vi "Analog Sensors.vi"() -> ()   [LabVIEW 2014]
uses:
  <vilib>/eio/EIONode/EIONode.xnode
  <vilib>/rvi/eio/common/nirviEmuTemplateMethod_errors.vi
panel:
  out "5V Reference":fxp<+/-,16,5>
  out "Throttle Percentage":fxp<+/-,33,17>
  out "Throttle Pot (V)":fxp<+/-,16,5>
  out "Rotation Rate (degrees/s)":fxp<+/-,64,33>
  out "Steering Wheel Angle (degrees)":fxp<+/-,48,32>
  out "ticks/count 4":u32
  out "ticks/count 3":u32
  out "ticks/count 2":u32
  out "ticks/count":u32
  in  "stop 2":bool
  out "SpeedZ":fxp<+/-,32,29>
  out "SpeedY":fxp<+/-,32,29>
  out "SpeedX":fxp<+/-,32,29>
  out "AccelZ (G)":fxp<+/-,42,25>
  out "AccelY (G)":fxp<+/-,42,25>
  out "AccelX (G)":fxp<+/-,42,25>
  in  "stop":bool
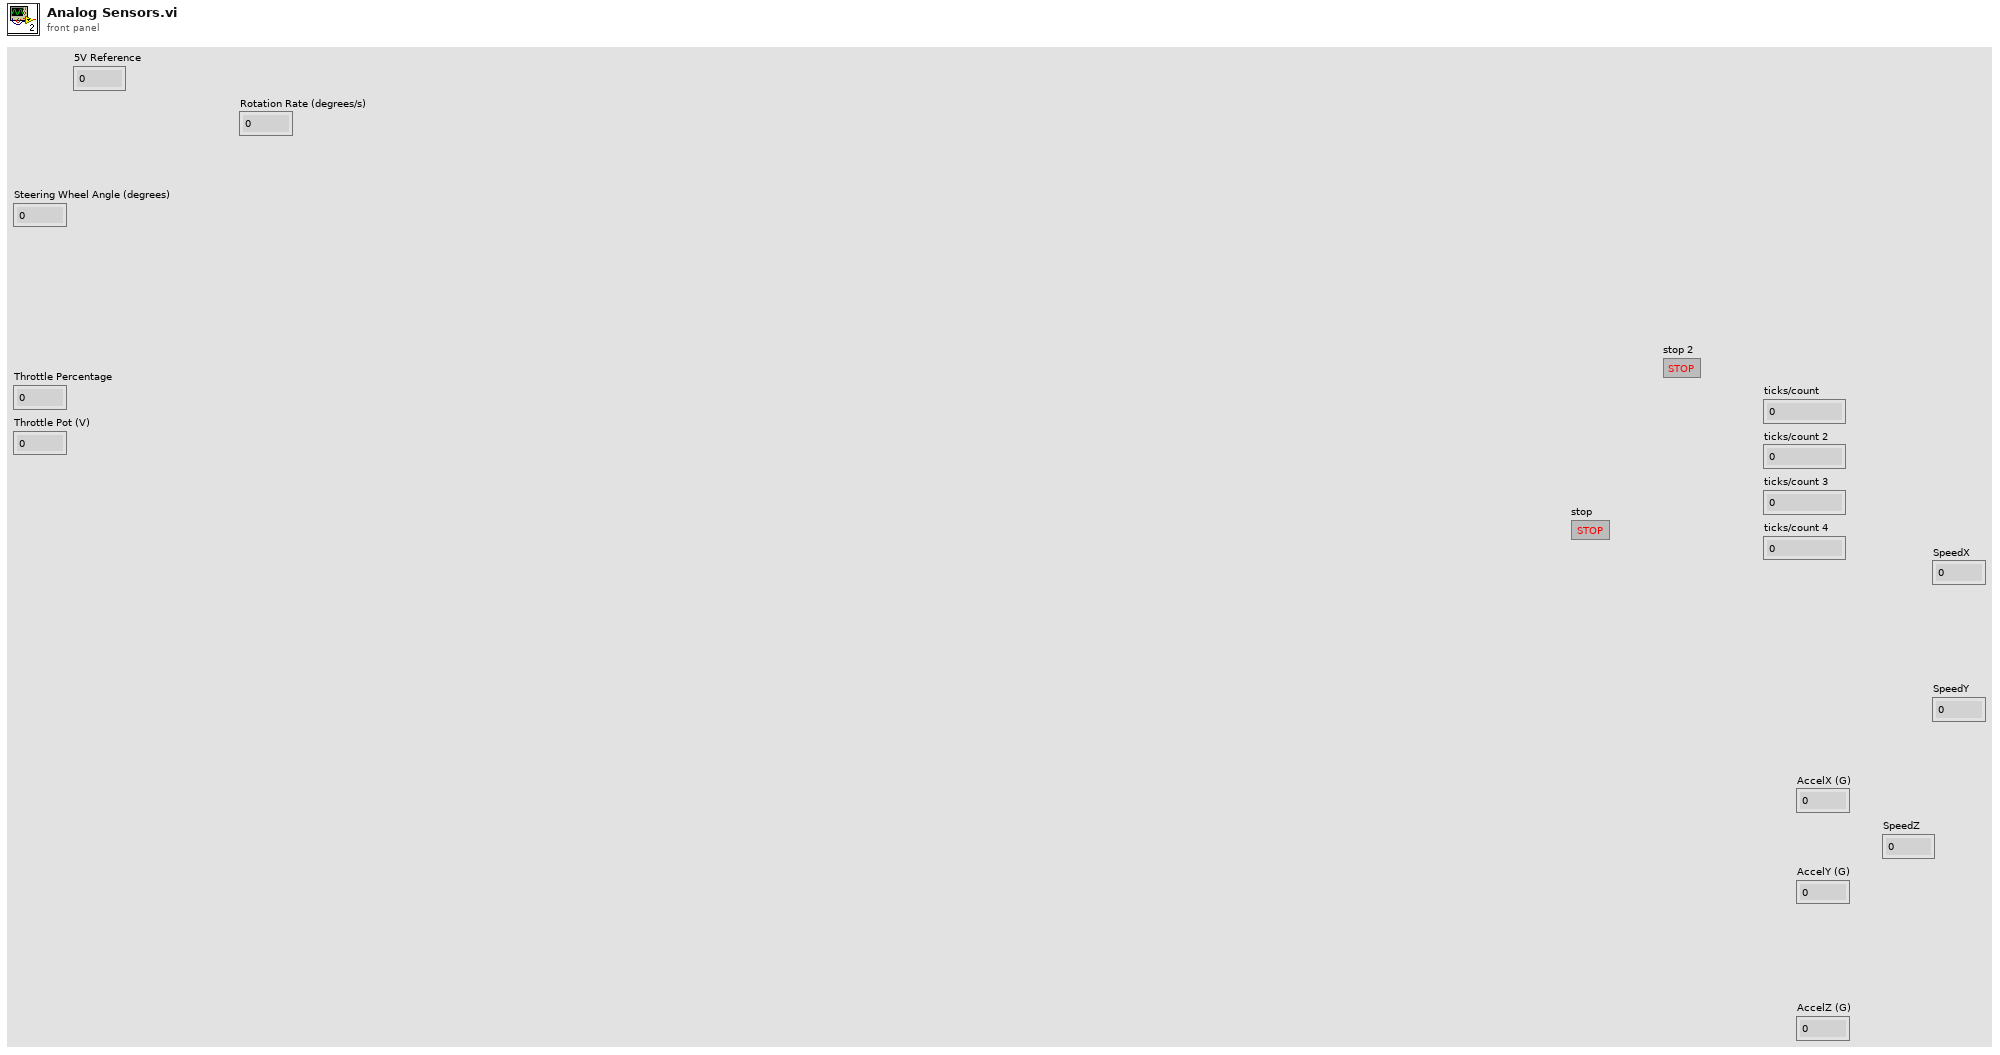
[diagram p1: front panel]
types:
  T1 = enum16{"Wheel Speed 1", "Wheel Speed 2", "Wheel Speed 3", "Wheel Speed 4"}
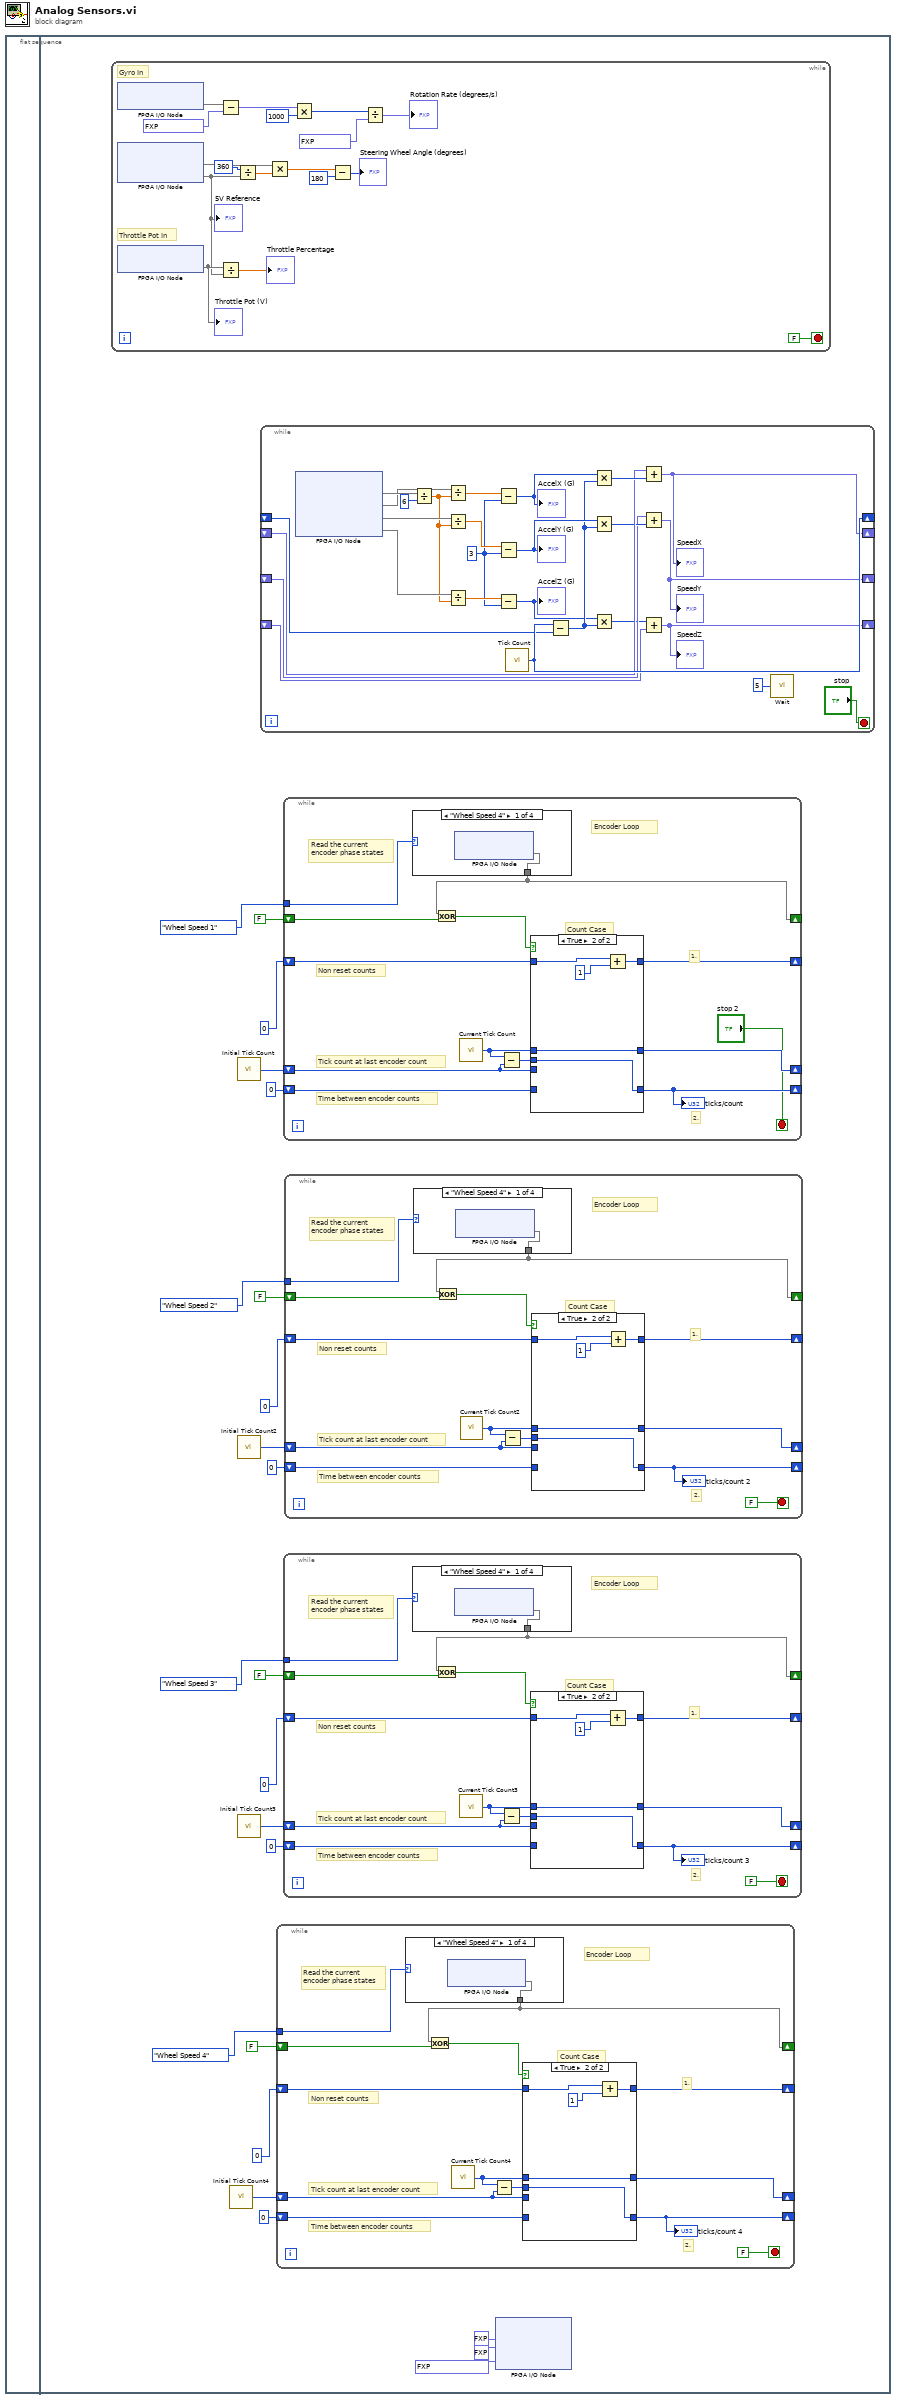
[diagram p0: block diagram]
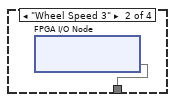
[diagram p2: hidden frame]
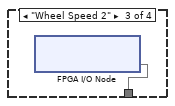
[diagram p3: hidden frame]
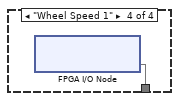
[diagram p4: hidden frame]
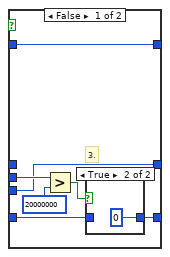
[diagram p5: hidden frame]
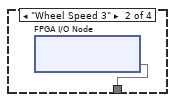
[diagram p7: hidden frame]
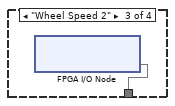
[diagram p8: hidden frame]
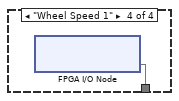
[diagram p9: hidden frame]
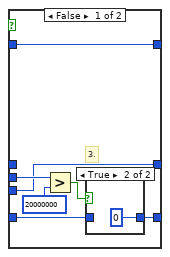
[diagram p10: hidden frame]
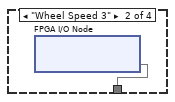
[diagram p12: hidden frame]
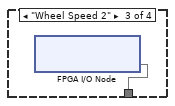
[diagram p13: hidden frame]
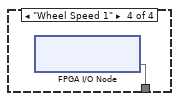
[diagram p14: hidden frame]
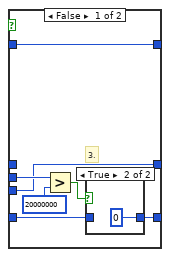
[diagram p15: hidden frame]
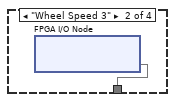
[diagram p17: hidden frame]
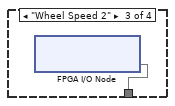
[diagram p18: hidden frame]
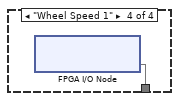
[diagram p19: hidden frame]
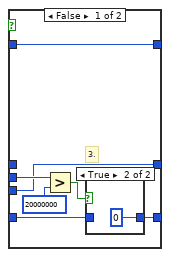
[diagram p20: hidden frame]
diagram:
  n1 = flat-sequence {
    frame #0 {
    }
    frame #1 {
      n2 = while {
        stop <- FALSE stop-if-true
        # "Throttle Pot In"
        # "Gyro In"
        n3 = xnode "FPGA I/O Node"() -> ("Analog In/AI6"=w34)  [unwired: 1 in, 1 out]
        n4 = xnode "FPGA I/O Node"() -> ("Analog In/AI0"=w39, "Analog In/AI1"=w26)  [unwired: 2 in, 2 out]
        "5V Reference" <- w26
        n5 = xnode "FPGA I/O Node"() -> ("Analog In/AI7"=w27)  [unwired: 1 in, 1 out]
        "Throttle Pot (V)" <- w27
        n6 = Subtract(x=w34, y=fxp<+/-,16,5> 1.22998046875) -> (x-y=w32:fxp<+/-,17,6>)
        n7 = Divide(x=w27, y=w26) -> (x/y=→"Throttle Percentage":dbl)
        n8 = Divide(x=i16 360, y=w26) -> (x/y=w38:dbl)
        n9 = Multiply(x=w39, y=w38) -> (x*y=w37:dbl)
        n10 = Multiply(x=w32, y=u16 1000) -> (x*y=w30:u16)
        n11 = Subtract(x=w37, y=u8 180) -> (x-y=→"Steering Wheel Angle (degrees)":u8)
        n12 = Divide(x=w30, y=fxp<+/-,33,22> 3.330078125) -> (x/y=→"Rotation Rate (degrees/s)":fxp<+/-,50,28>)
      }
      n13 = call "Initial Tick Count4"() -> ("Tick Count(Ticks)"=w6:u32)
      n14 = call "Initial Tick Count"() -> ("Tick Count(Ticks)"=w21:u32)
      n15 = call "Initial Tick Count3"() -> ("Tick Count(Ticks)"=w11:u32)
      n16 = call "Initial Tick Count2"() -> ("Tick Count(Ticks)"=w16:u32)
      n17 = while {
        shift-right: [w179] -> _
        shift-left: _ -> [w178]
        shift-right: [w171] -> _
        shift-left: _ -> [w172]
        shift-right: [w168] -> _
        shift-left: _ -> [w169]
        shift-right: [w165] -> _
        shift-left: _ -> [w166]
        stop <- "stop" stop-if-true
        w180 = i8 3 ("y")
        n18 = xnode "FPGA I/O Node"() -> ("Analog In/AI2"=w187, "Analog In/AI3"=w186, "Analog In/AI4"=w185, "Analog In/AI5"=w183)  [unwired: 4 in, 4 out]
        n19 = Divide(x=w187, y=i8 6) -> (x/y=w182:dbl)
        n20 = Divide(x=w186, y=w182) -> (x/y=w188:dbl)
        n21 = Divide(x=w185, y=w182) -> (x/y=w184:dbl)
        n22 = Divide(x=w183, y=w182) -> (x/y=w181:dbl)
        n23 = Subtract(x=w188, y=w180) -> (x-y=w177:i8)
        "AccelX (G)" <- w177
        n24 = Subtract(x=w184, y=w180) -> (x-y=w176:i8)
        "AccelY (G)" <- w176
        n25 = Subtract(x=w181, y=w180) -> (x-y=w174:i8)
        "AccelZ (G)" <- w174
        n26 = call "Tick Count"() -> ("Tick Count(uSec)"=w179:u32)
        n27 = Subtract(x=w179, y=w178) -> (x-y=w175:u32)
        n28 = Multiply(x=w177, y=w175) -> (x*y=w173:u32)
        n29 = Multiply(x=w176, y=w175) -> (x*y=w170:u32)
        n30 = Multiply(x=w174, y=w175) -> (x*y=w167:u32)
        n31 = Add(x=w172, y=w173) -> (x+y=w171:fxp<+/-,32,29>)
        "SpeedX" <- w171
        n32 = Add(x=w169, y=w170) -> (x+y=w168:fxp<+/-,32,29>)
        "SpeedY" <- w168
        n33 = Add(x=w167, y=w166) -> (x+y=w165:fxp<+/-,32,29>)
        "SpeedZ" <- w165
        n34 = call "Wait"("Count(mSec)"=u8 5) -> ()  [unwired: 1 out]
      }
      n35 = while {
        shift-right: [w41] -> _
        shift-left: FALSE ("Encoder Phase A") -> [w53]
        shift-right: [w52] -> _
        shift-left: w6 -> [w46]
        shift-right: [w51] -> _
        shift-left: u32 0 -> [w50]
        shift-right: [w47] -> _
        shift-left: 0 ("Reset Position Value") -> [w48]
        tunnel: T1."Wheel Speed 4" ("Sensor Number") -> [w42]
        stop <- FALSE stop-if-true
        # "Encoder Loop"
        # "Count Case"
        # "2."
        # "1."
        # "Read the current\nencoder phase states"
        # "Non reset counts"
        # "Time between encoder counts"
        # "Tick count at last encoder count"
        n36 = case shown="\"Wheel Speed 4\"" w42 {
          tunnel: [w54 w55 w56 w57] -> w41
          frame "Wheel Speed 4" {
            n37 = xnode "FPGA I/O Node"() -> ("Mod1/DIO4"=w54)  [unwired: 1 in, 1 out]
          }
          frame "Wheel Speed 3" {
            n38 = xnode "FPGA I/O Node"() -> ("Mod1/DIO2"=w55)  [unwired: 1 in, 1 out]
          }
          frame "Wheel Speed 2" {
            n39 = xnode "FPGA I/O Node"() -> ("Mod1/DIO1"=w56)  [unwired: 1 in, 1 out]
          }
          frame "Wheel Speed 1" {
            n40 = xnode "FPGA I/O Node"() -> ("Mod1/DIO0"=w57)  [unwired: 1 in, 1 out]
          }
        }
        n41 = Exclusive Or(1:w53, 2:w41) -> (0:w43:bool)
        n42 = call "Current Tick Count4"() -> ("Tick Count(Ticks)"=w44:u32)
        n43 = Subtract(x=w44, y=w46) -> (x-y=w45:u32)
        n44 = case shown="True" w43 {
          tunnel: [w58 w69] -> w52
          tunnel: w46 -> [w58 _]
          tunnel: [w61 w68] -> w51
          tunnel: w50 -> [w60 _]
          tunnel: [w64 w71] -> w47
          tunnel: w48 -> [w64 w70]
          tunnel: w45 -> [w59 w68]
          tunnel: w44 -> [_ w69]
          frame False {
            # "3."
            n45 = Greater?(x=w59, y=20000000 ("x")) -> (0:w62:bool)
            n46 = case shown="True" w62 {
              tunnel: [w65 u32 0] -> w61
              tunnel: w60 -> [w65 _]
              frame False {
              }
              frame True {
              }
            }
          }
          frame True {
            n47 = Add(x=w70, y=1 ("16 bit")) -> (x+y=w71:i32)
          }
        }
        "ticks/count 4" <- w51
      }
      n48 = while {
        shift-right: [w135] -> _
        shift-left: FALSE ("Encoder Phase A") -> [w146]
        shift-right: [w145] -> _
        shift-left: w21 -> [w140]
        shift-right: [w144] -> _
        shift-left: u32 0 -> [w143]
        shift-right: [w141] -> _
        shift-left: 0 ("Reset Position Value") -> [w142]
        tunnel: T1."Wheel Speed 1" ("Sensor Number") -> [w136]
        stop <- "stop 2" stop-if-true
        # "Encoder Loop"
        # "Count Case"
        # "2."
        # "1."
        # "Read the current\nencoder phase states"
        # "Non reset counts"
        # "Time between encoder counts"
        # "Tick count at last encoder count"
        n49 = case shown="\"Wheel Speed 4\"" w136 {
          tunnel: [w147 w148 w149 w150] -> w135
          frame "Wheel Speed 4" {
            n50 = xnode "FPGA I/O Node"() -> ("Mod1/DIO4"=w147)  [unwired: 1 in, 1 out]
          }
          frame "Wheel Speed 3" {
            n51 = xnode "FPGA I/O Node"() -> ("Mod1/DIO2"=w148)  [unwired: 1 in, 1 out]
          }
          frame "Wheel Speed 2" {
            n52 = xnode "FPGA I/O Node"() -> ("Mod1/DIO1"=w149)  [unwired: 1 in, 1 out]
          }
          frame "Wheel Speed 1" {
            n53 = xnode "FPGA I/O Node"() -> ("Mod1/DIO0"=w150)  [unwired: 1 in, 1 out]
          }
        }
        n54 = Exclusive Or(1:w146, 2:w135) -> (0:w137:bool)
        n55 = call "Current Tick Count"() -> ("Tick Count(Ticks)"=w138:u32)
        n56 = Subtract(x=w138, y=w140) -> (x-y=w139:u32)
        n57 = case shown="True" w137 {
          tunnel: [w151 w162] -> w145
          tunnel: w140 -> [w151 _]
          tunnel: [w154 w161] -> w144
          tunnel: w143 -> [w153 _]
          tunnel: [w157 w164] -> w141
          tunnel: w142 -> [w157 w163]
          tunnel: w139 -> [w152 w161]
          tunnel: w138 -> [_ w162]
          frame False {
            # "3."
            n58 = Greater?(x=w152, y=20000000 ("x")) -> (0:w155:bool)
            n59 = case shown="True" w155 {
              tunnel: [w158 u32 0] -> w154
              tunnel: w153 -> [w158 _]
              frame False {
              }
              frame True {
              }
            }
          }
          frame True {
            n60 = Add(x=w163, y=1 ("16 bit")) -> (x+y=w164:i32)
          }
        }
        "ticks/count" <- w144
      }
      n61 = while {
        shift-right: [w72] -> _
        shift-left: FALSE ("Encoder Phase A") -> [w84]
        shift-right: [w83] -> _
        shift-left: w11 -> [w77]
        shift-right: [w82] -> _
        shift-left: u32 0 -> [w81]
        shift-right: [w78] -> _
        shift-left: 0 ("Reset Position Value") -> [w79]
        tunnel: T1."Wheel Speed 3" ("Sensor Number") -> [w73]
        stop <- FALSE stop-if-true
        # "Encoder Loop"
        # "Count Case"
        # "2."
        # "1."
        # "Read the current\nencoder phase states"
        # "Non reset counts"
        # "Time between encoder counts"
        # "Tick count at last encoder count"
        n62 = case shown="\"Wheel Speed 4\"" w73 {
          tunnel: [w85 w86 w87 w88] -> w72
          frame "Wheel Speed 4" {
            n63 = xnode "FPGA I/O Node"() -> ("Mod1/DIO4"=w85)  [unwired: 1 in, 1 out]
          }
          frame "Wheel Speed 3" {
            n64 = xnode "FPGA I/O Node"() -> ("Mod1/DIO2"=w86)  [unwired: 1 in, 1 out]
          }
          frame "Wheel Speed 2" {
            n65 = xnode "FPGA I/O Node"() -> ("Mod1/DIO1"=w87)  [unwired: 1 in, 1 out]
          }
          frame "Wheel Speed 1" {
            n66 = xnode "FPGA I/O Node"() -> ("Mod1/DIO0"=w88)  [unwired: 1 in, 1 out]
          }
        }
        n67 = Exclusive Or(1:w84, 2:w72) -> (0:w74:bool)
        n68 = call "Current Tick Count3"() -> ("Tick Count(Ticks)"=w75:u32)
        n69 = Subtract(x=w75, y=w77) -> (x-y=w76:u32)
        n70 = case shown="True" w74 {
          tunnel: [w89 w100] -> w83
          tunnel: w77 -> [w89 _]
          tunnel: [w92 w99] -> w82
          tunnel: w81 -> [w91 _]
          tunnel: [w95 w102] -> w78
          tunnel: w79 -> [w95 w101]
          tunnel: w76 -> [w90 w99]
          tunnel: w75 -> [_ w100]
          frame False {
            # "3."
            n71 = Greater?(x=w90, y=20000000 ("x")) -> (0:w93:bool)
            n72 = case shown="True" w93 {
              tunnel: [w96 u32 0] -> w92
              tunnel: w91 -> [w96 _]
              frame False {
              }
              frame True {
              }
            }
          }
          frame True {
            n73 = Add(x=w101, y=1 ("16 bit")) -> (x+y=w102:i32)
          }
        }
        "ticks/count 3" <- w82
      }
      n74 = while {
        shift-right: [w103] -> _
        shift-left: FALSE ("Encoder Phase A") -> [w115]
        shift-right: [w114] -> _
        shift-left: w16 -> [w108]
        shift-right: [w113] -> _
        shift-left: u32 0 -> [w112]
        shift-right: [w109] -> _
        shift-left: 0 ("Reset Position Value") -> [w110]
        tunnel: T1."Wheel Speed 2" ("Sensor Number") -> [w104]
        stop <- FALSE stop-if-true
        # "Encoder Loop"
        # "Count Case"
        # "2."
        # "1."
        # "Read the current\nencoder phase states"
        # "Non reset counts"
        # "Time between encoder counts"
        # "Tick count at last encoder count"
        n75 = case shown="\"Wheel Speed 4\"" w104 {
          tunnel: [w116 w117 w118 w119] -> w103
          frame "Wheel Speed 4" {
            n76 = xnode "FPGA I/O Node"() -> ("Mod1/DIO4"=w116)  [unwired: 1 in, 1 out]
          }
          frame "Wheel Speed 3" {
            n77 = xnode "FPGA I/O Node"() -> ("Mod1/DIO2"=w117)  [unwired: 1 in, 1 out]
          }
          frame "Wheel Speed 2" {
            n78 = xnode "FPGA I/O Node"() -> ("Mod1/DIO1"=w118)  [unwired: 1 in, 1 out]
          }
          frame "Wheel Speed 1" {
            n79 = xnode "FPGA I/O Node"() -> ("Mod1/DIO0"=w119)  [unwired: 1 in, 1 out]
          }
        }
        n80 = Exclusive Or(1:w115, 2:w103) -> (0:w105:bool)
        n81 = call "Current Tick Count2"() -> ("Tick Count(Ticks)"=w106:u32)
        n82 = Subtract(x=w106, y=w108) -> (x-y=w107:u32)
        n83 = case shown="True" w105 {
          tunnel: [w120 w131] -> w114
          tunnel: w108 -> [w120 _]
          tunnel: [w123 w130] -> w113
          tunnel: w112 -> [w122 _]
          tunnel: [w126 w133] -> w109
          tunnel: w110 -> [w126 w132]
          tunnel: w107 -> [w121 w130]
          tunnel: w106 -> [_ w131]
          frame False {
            # "3."
            n84 = Greater?(x=w121, y=20000000 ("x")) -> (0:w124:bool)
            n85 = case shown="True" w124 {
              tunnel: [w127 u32 0] -> w123
              tunnel: w122 -> [w127 _]
              frame False {
              }
              frame True {
              }
            }
          }
          frame True {
            n86 = Add(x=w132, y=1 ("16 bit")) -> (x+y=w133:i32)
          }
        }
        "ticks/count 2" <- w113
      }
      n87 = xnode "FPGA I/O Node"("Mod3/AO0"=fxp<+/-,20,5> 3.0, "Mod3/AO1"=fxp<+/-,20,5> 5.0, "Mod3/AO2"=fxp<+/-,20,5> 3.29998779296875) -> ()  [unwired: 3 in, 3 out]
    }
  }
